vi "Coord window-Globals.vi"() -> ()   [LabVIEW 2020]
uses:
  Typedefs/Coordinate list window refs.ctl
  <vilib>/Utility/miscctls.llb/LVRowAndColumnTypeDef.ctl
panel:
  in  "Item Names + exp params":string[][](array[string])
  in  "Column names header name":string="COLUMN NAMES"
  in  "Parameters header name":string="PARAMETERS"
  in  "Coordinates header name":string="COORDINATES & INFO"
  in  "FOV (during experiments)":sgl
  in  "Zoom (during experiments)":i8
  in  "Motor dot size":i16=2
  out "Normalised Effective FOV":T1
  in  "Motor coordinates colour":u32(colorbox)=6618880
  out "Cell position":T2
  in  "Column Sizes":u32[](array[numeric])=[54, 54, 54, 135, 135, 135, 135, 135, 135, 135, 135, 135, 135, 135, 135, 135, 135, 135, 135, 135, 135, 135, 135, 135, 135, 135, 135, 135, 135, 135, 135]
  in  "Key focus?":bool
  in  "Bring to front":bool
  in  "Window is open":bool
  in  "Save as new file":bool=TRUE
  in  "Coord file loaded":bool
  in  "Coordinate list window refs":T3
  out "Previous values":string[][](array[string])
  in  "Picture map range":cluster{"Min (um)":dbl, "Max (um)":dbl}={"Min (um)"=-20000.0, "Max (um)"=20000.0}
  in  "Last accessed coordinates file":path
  # "<--- This is the index of the cell the user right clicked on."
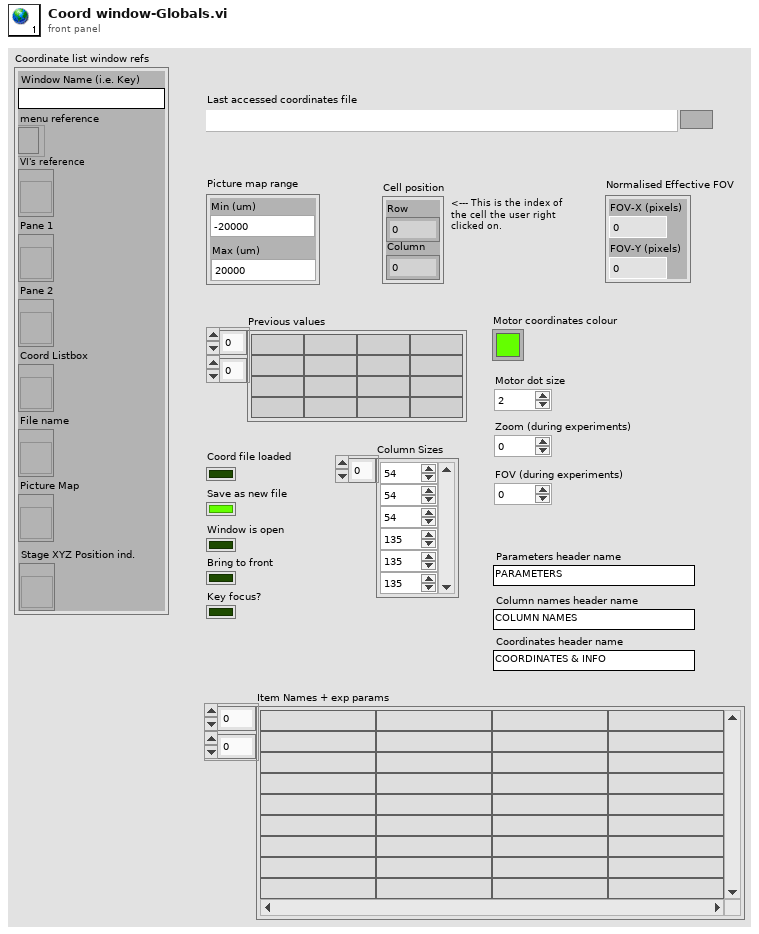
[diagram p1: front panel]
types:
  T1 = cluster{"FOV-X (pixels)":i16, "FOV-Y (pixels)":i16}
  T2 = typedef "LVRowAndColumnTypeDef.ctl" = cluster{"Row":i32, "Column":i32}
  T3 = typedef "Coordinate list window refs.ctl" = cluster{"Window Name (i.e. Key)":string, "menu reference":refnum<k9>, "VI's reference":refnum<vi>, "Pane 1":refnum<vi>, "Pane 2":refnum<vi>, "Coord Listbox":refnum<vi>, "File name":refnum<vi>, "Picture Map":refnum<vi>, "Stage XYZ Position ind.":refnum<vi>}
diagram:
